vi "sub_vi.vi"() -> ()   [LabVIEW 2025]
panel:
  out "X":dbl
  in  "B":dbl
  in  "X":dbl
  in  "A":dbl
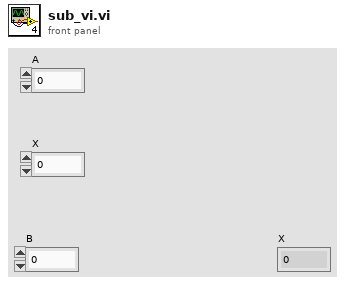
[diagram p1: front panel]
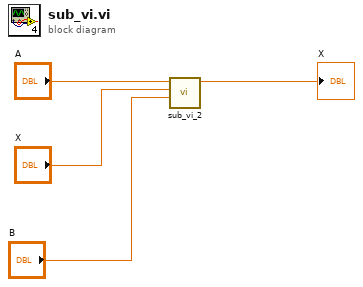
[diagram p0: block diagram]
diagram:
  n1 = call "sub_vi_2.vi"("B"="B", "X"="X", "A"="A") -> ("Numeric"=→"X":dbl)  [unwired: 8 in]
